vi "Get User Interface VI.vi"(8 "error in (no error)":errorcluster, 11 "UDPlog Transfer Rx User Interface in":refnum<class "UDPlog Transfer Rx User Interface.lvclass">) -> (0 "error out":errorcluster, 2 "user interface vi":refnum<vi>, 3 "UDPlog Transfer Rx User Interface out":refnum<class "UDPlog Transfer Rx User Interface.lvclass">)   [LabVIEW 2023, in "UDPlog.lvlib" / "UDPlog Transfer Rx User Interface.lvclass"]
uses:
  UDPlog Transfer Rx User Interface.lvclass
  UDPlog Transfer Rx User Interface.lvclass/UDPlog Transfer Rx User Interface.ctl
  User Interface.vi
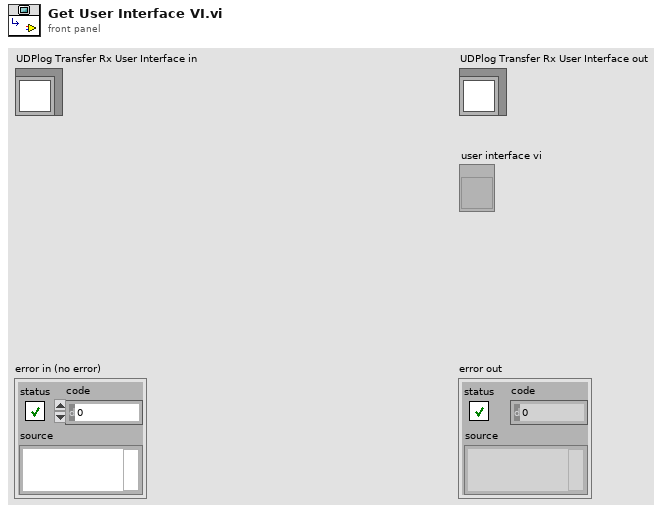
[diagram p1: front panel]
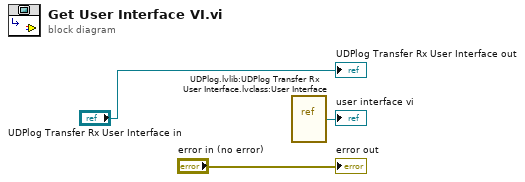
[diagram p0: block diagram]
diagram:
  n1 = vi-ref "UDPlog.lvlib:UDPlog Transfer Rx User Interface.lvclass:User Interface.vi"() -> (→"user interface vi":refnum<vi>)
  "error out" <- "error in (no error)"
  "UDPlog Transfer Rx User Interface out" <- "UDPlog Transfer Rx User Interface in"
